vi "Set_Read_Temperature_SP.vi"(7 "error in (no error)":errorcluster, 9 "setpoint":dbl, 10 "Omega CN9600 series.lvclass":refnum<class "Omega CN9600 series.lvclass">) -> (0 "error out":errorcluster, 2 "actual setpoint":dbl, 3 "Omega CN9600 series.lvclass 2":refnum<class "Omega CN9600 series.lvclass">)   [LabVIEW 2014, in "Omega CN9600 series.lvclass"]
uses:
  Omega CN9600 series.lvclass
  Omega CN9600 series.lvclass/Omega CN9600 series.ctl
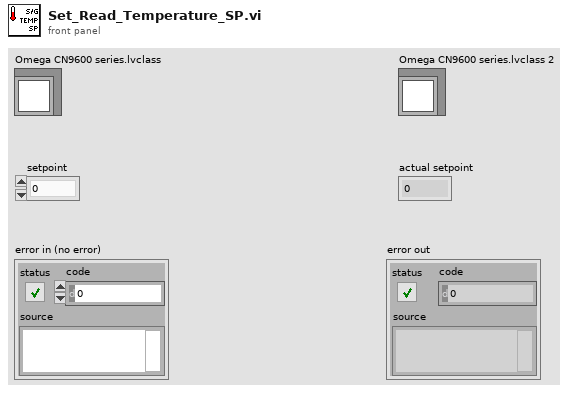
[diagram p1: front panel]
types:
  T1 = typedef "Omega CN9600 series.lvclass/Serial_Config_Omega.ctl" = cluster{"Baud":u32, "Flow Ctl":u16, "Parity":u16, "Address":u8, "VISA resource name":refnum<visa-resource-name>}
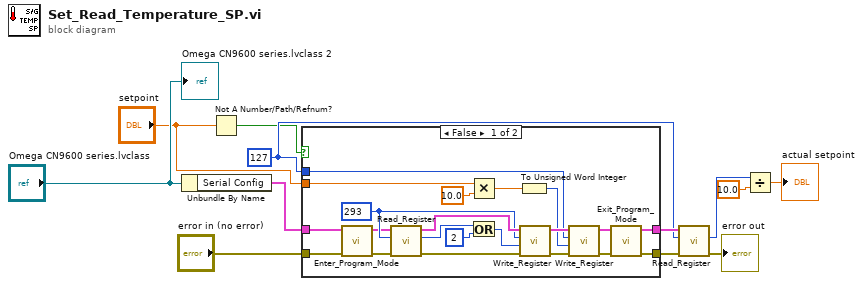
[diagram p0: block diagram]
diagram:
  w4 = u16 127 ("Address")
  n1 = Unbundle By Name("Omega CN9600 series.lvclass") -> ("Serial Config"=w8:T1)
  n2 = Not A Number/Path/Refnum?(number/path/refnum="setpoint") -> (NaN/Path/Refnum?=w2:bool)
  n3 = case shown="False" w2 {
    tunnel: "setpoint" -> [w25 _]
    tunnel: w8 -> [w21 w35]
    tunnel: "error in (no error)" -> [w20 w34]
    tunnel: [w16 w35] -> w6
    tunnel: [w14 w34] -> w1
    tunnel: w4 -> [w13 _]
    frame False {
      w28 = u16 293 ("Address")
      n4 = call "Enter_Program_Mode.vi"("error in (no error)"=w20, "Serial Config"=w21) -> ("error out"=w19:errorcluster, "Serial Config out"=w18:T1)  [unwired: 8 in]
      n5 = call "Read_Register.vi"("error in (no error)"=w19, "Address"=w28, "Serial Config"=w18) -> ("error out"=w26:errorcluster, "Value"=w32:u16, "Serial Config out"=w33:T1)  [unwired: 6 in]
      n6 = Multiply(x=w25, y=10.0) -> (x*y=w23:dbl)
      n7 = Or(x=w32, y=u16 2) -> (x .or. y?=w30:u16)
      n8 = To Unsigned Word Integer(number=w23) -> (unsigned 16bit integer=w22:u16)
      n9 = call "Write_Register.vi"("error in (no error)"=w26, "Value"=w30, "Address"=w28, "Serial Config"=w33) -> ("error out"=w27:errorcluster, "Serial Config out"=w29:T1)  [unwired: 6 in]
      n10 = call "Write_Register.vi"("error in (no error)"=w27, "Value"=w22, "Address"=w13, "Serial Config"=w29) -> ("error out"=w15:errorcluster, "Serial Config out"=w17:T1)  [unwired: 6 in]
      n11 = call "Exit_Program_Mode.vi"("error in (no error)"=w15, "Serial Config"=w17) -> ("error out"=w14:errorcluster, "Serial Config out"=w16:T1)  [unwired: 8 in]
    }
    frame True {
    }
  }
  n12 = call "Read_Register.vi"("error in (no error)"=w1, "Address"=w4, "Serial Config"=w6) -> ("error out"=→"error out":errorcluster, "Value"=w10:u16)  [unwired: 6 in, 1 out]
  n13 = Divide(x=w10, y=10.0) -> (x/y=→"actual setpoint":dbl)
  "Omega CN9600 series.lvclass 2" <- "Omega CN9600 series.lvclass"
